vi "Meal Calculator.vi"() -> ()   [LabVIEW 2010]
panel:
  in  "Tax Percentage":dbl
  in  "Side":enum16{"Onion Rings", "Salad"}(ring)
  in  "Drink":enum16{"Water", "Juice"}(ring)
  out "Total Price":dbl format="%#.2g"
  in  "# of Sides":i32
  in  "# of Drinks":i32
  in  "# of Mains":i32
  in  "Main":enum16{"Chicken Nuggets", "Chicken Sandwich"}(ring)
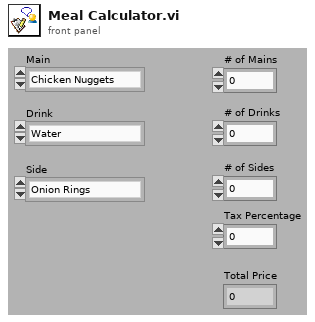
[diagram p1: front panel]
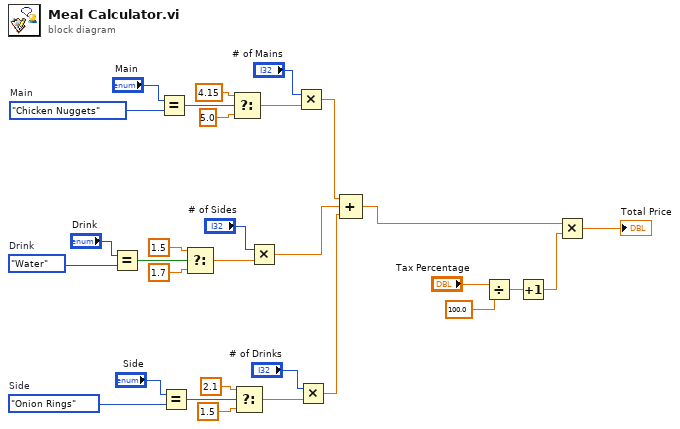
[diagram p0: block diagram]
diagram:
  w5 = enum16{"Onion Rings", "Salad"}."Onion Rings"  # Side
  w8 = enum16{"Water", "Juice"}."Water"  # Drink
  w13 = enum16{"Chicken Nuggets", "Chicken Sandwich"}."Chicken Nuggets"  # Main
  n1 = Equal?(x="Drink", y=w8) -> (x = y?=w19:bool)
  n2 = Equal?(x="Main", y=w13) -> (x = y?=w25:bool)
  n3 = Equal?(x="Side", y=w5) -> (x = y?=w17:bool)
  n4 = Select(t=1.5, s=w19, f=1.7) -> (s? t:f=w18:dbl)
  n5 = Select(t=4.15, s=w25, f=5.0) -> (s? t:f=w22:dbl)
  n6 = Select(t=2.1, s=w17, f=1.5) -> (s? t:f=w14:dbl)
  n7 = Multiply(x="# of Sides", y=w18) -> (x*y=w29:dbl)
  n8 = Multiply(x="# of Mains", y=w22) -> (x*y=w30:dbl)
  n9 = Multiply(x="# of Drinks", y=w14) -> (x*y=w28:dbl)
  n10 = Compound Arithmetic op=ADD(w30, w29, w28) -> (w27:dbl)
  n11 = Divide(x="Tax Percentage", y=100.0) -> (x/y=w1:dbl)
  n12 = Increment(x=w1) -> (x+1=w26:dbl)
  n13 = Multiply(x=w27, y=w26) -> (x*y=→"Total Price":dbl)
